vi "Batch Data Extractor.vi"(8 "Error In":errorcluster, 9 "Batch Data":variant[][](array[variant])=[[variant]], 10 "Batch Label":string, 11 "Author ID":i32) -> (0 "Error Out":errorcluster, 2 "Exists?":bool, 3 "Batch Information":cluster{"Batch Label":string, "Batch ID":i32})   [LabVIEW 2020]
uses:
  <vilib>/addons/database/_DB Variant To Data/Database Variant To Data.xnode
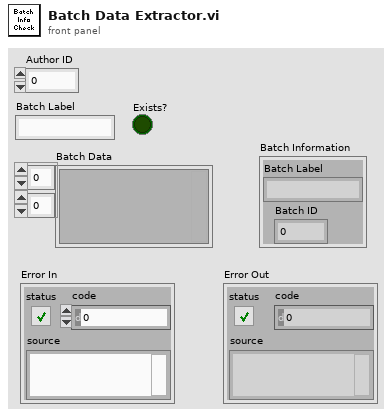
[diagram p1: front panel]
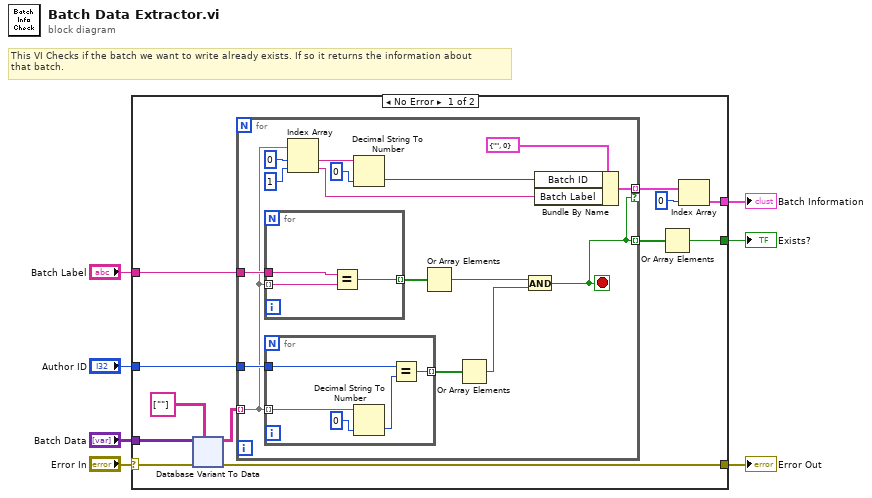
[diagram p0: block diagram]
diagram:
  # "This VI Checks if the batch we want to write already exists. If so it returns the information about\nthat batch."
  n1 = case shown="No Error" "Error In" {
    selector: "Error In" -> [w15 w88]
    tunnel: "Batch Data" -> [w16 _]
    tunnel: "Batch Label" -> [w14 _]
    tunnel: [w12 _] -> w4
    tunnel: [w13 w88] -> w3
    tunnel: [w9 _] -> w2
    tunnel: "Author ID" -> [w8 _]
    frame No Error {
      n2 = xnode "Database Variant To Data"("database variant"=w16, "error in (no error)"=w15, "type"=string[][] [[""]] ("columns")) -> ("data"=w17:string[][], "error out"=w13:errorcluster)
      n3 = for {
        tunnel: w17 -> [w24] mode=indexing
        tunnel: w14 -> [w35]
        tunnel: [w20] -> w18 mode=indexing
        tunnel: [w26] -> w11 mode=indexing if=w20
        tunnel: w8 -> [w25]
        stop <- w20 stop-if-true
        n4 = for {
          tunnel: w24 -> [w42] mode=indexing
          tunnel: w35 -> [w43]
          tunnel: [w41] -> w34 mode=indexing
          n5 = Equal?(x=w43, y=w42) -> (x = y?=w41:bool)
        }
        n6 = for {
          tunnel: w24 -> [w37] mode=indexing
          tunnel: w25 -> [w40]
          tunnel: [w39] -> w23 mode=indexing
          n7 = Decimal String To Number(string=w37, default (0L)=0 ("default (0 I32)")) -> (number=w36:i32)  [unwired: 1 in, 1 out]
          n8 = Equal?(x=w40, y=w36) -> (x = y?=w39:bool)
        }
        n9 = Index Array(array=w24, index #1=0 ("index"), index #2=1 ("index")) -> (element #1=w31:string, element #2=w28:string)
        n10 = Decimal String To Number(string=w31, default (0L)=0 ("default (0 I32)")) -> (number=w27:i32)  [unwired: 1 in, 1 out]
        n11 = Or Array Elements(Boolean array=w34) -> (logical OR=w22:bool)
        n12 = Or Array Elements(Boolean array=w23) -> (logical OR=w21:bool)
        n13 = And(x=w22, y=w21) -> (x .and. y?=w20:bool)
        n14 = Bundle By Name(cluster=cluster{"Batch Label":string, "Batch ID":i32} {"Batch Label"="", "Batch ID"=0} ("output cluster"), "Batch ID"=w27, "Batch Label"=w28) -> (w26:cluster{"Batch Label":string, "Batch ID":i32})
      }
      n15 = Or Array Elements(Boolean array=w18) -> (logical OR=w12:bool)
      n16 = Index Array(array=w11, index=0) -> (element=w9:cluster{"Batch Label":string, "Batch ID":i32})
    }
    frame Error {
    }
  }
  "Exists?" <- w4
  "Error Out" <- w3
  "Batch Information" <- w2
